vi "Periodic Tasks.vi"(0 "error in":errorcluster) -> ()   [LabVIEW 2020]
doc: "All TeleOperated, Autonomous, and Test controller logic are located here. Sensor reads and actuator commands are run inside of parallel loops. Most FRC 4265 code should be placed here."
uses:
  GlobalMiscellaneous.vi
  GlobalDriverStationData.vi
  GlobalAutonomous.vi
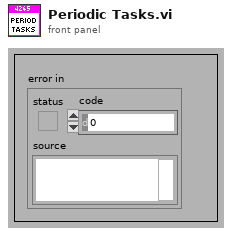
[diagram p1: front panel]
types:
  T1 = typedef "WPI_DriverStationRobotMode2.ctl" = enum16{"Autonomous Disabled", "Autonomous Enabled", "Teleop Disabled", "Teleop Enabled", "Disconnected", "Finish", "Test Disabled", "Test Enabled", "Emergency Stopped"}
  T2 = cluster{"Auto Error Out":errorcluster, "Drive Advance":bool, "Drive Step":i32, "Manipulator Step":i32, "Manipulator Advance":bool}
  T3 = cluster{"Auto Error":errorcluster, "Drive Advance":bool, "Drive Step":i32, "Manipulator Step":i32, "Manipulator Advance":bool}
  T4 = enum16{"Stowed", "Balancing", "Scoring", "Hoppering", "Ground", "Shelf"}
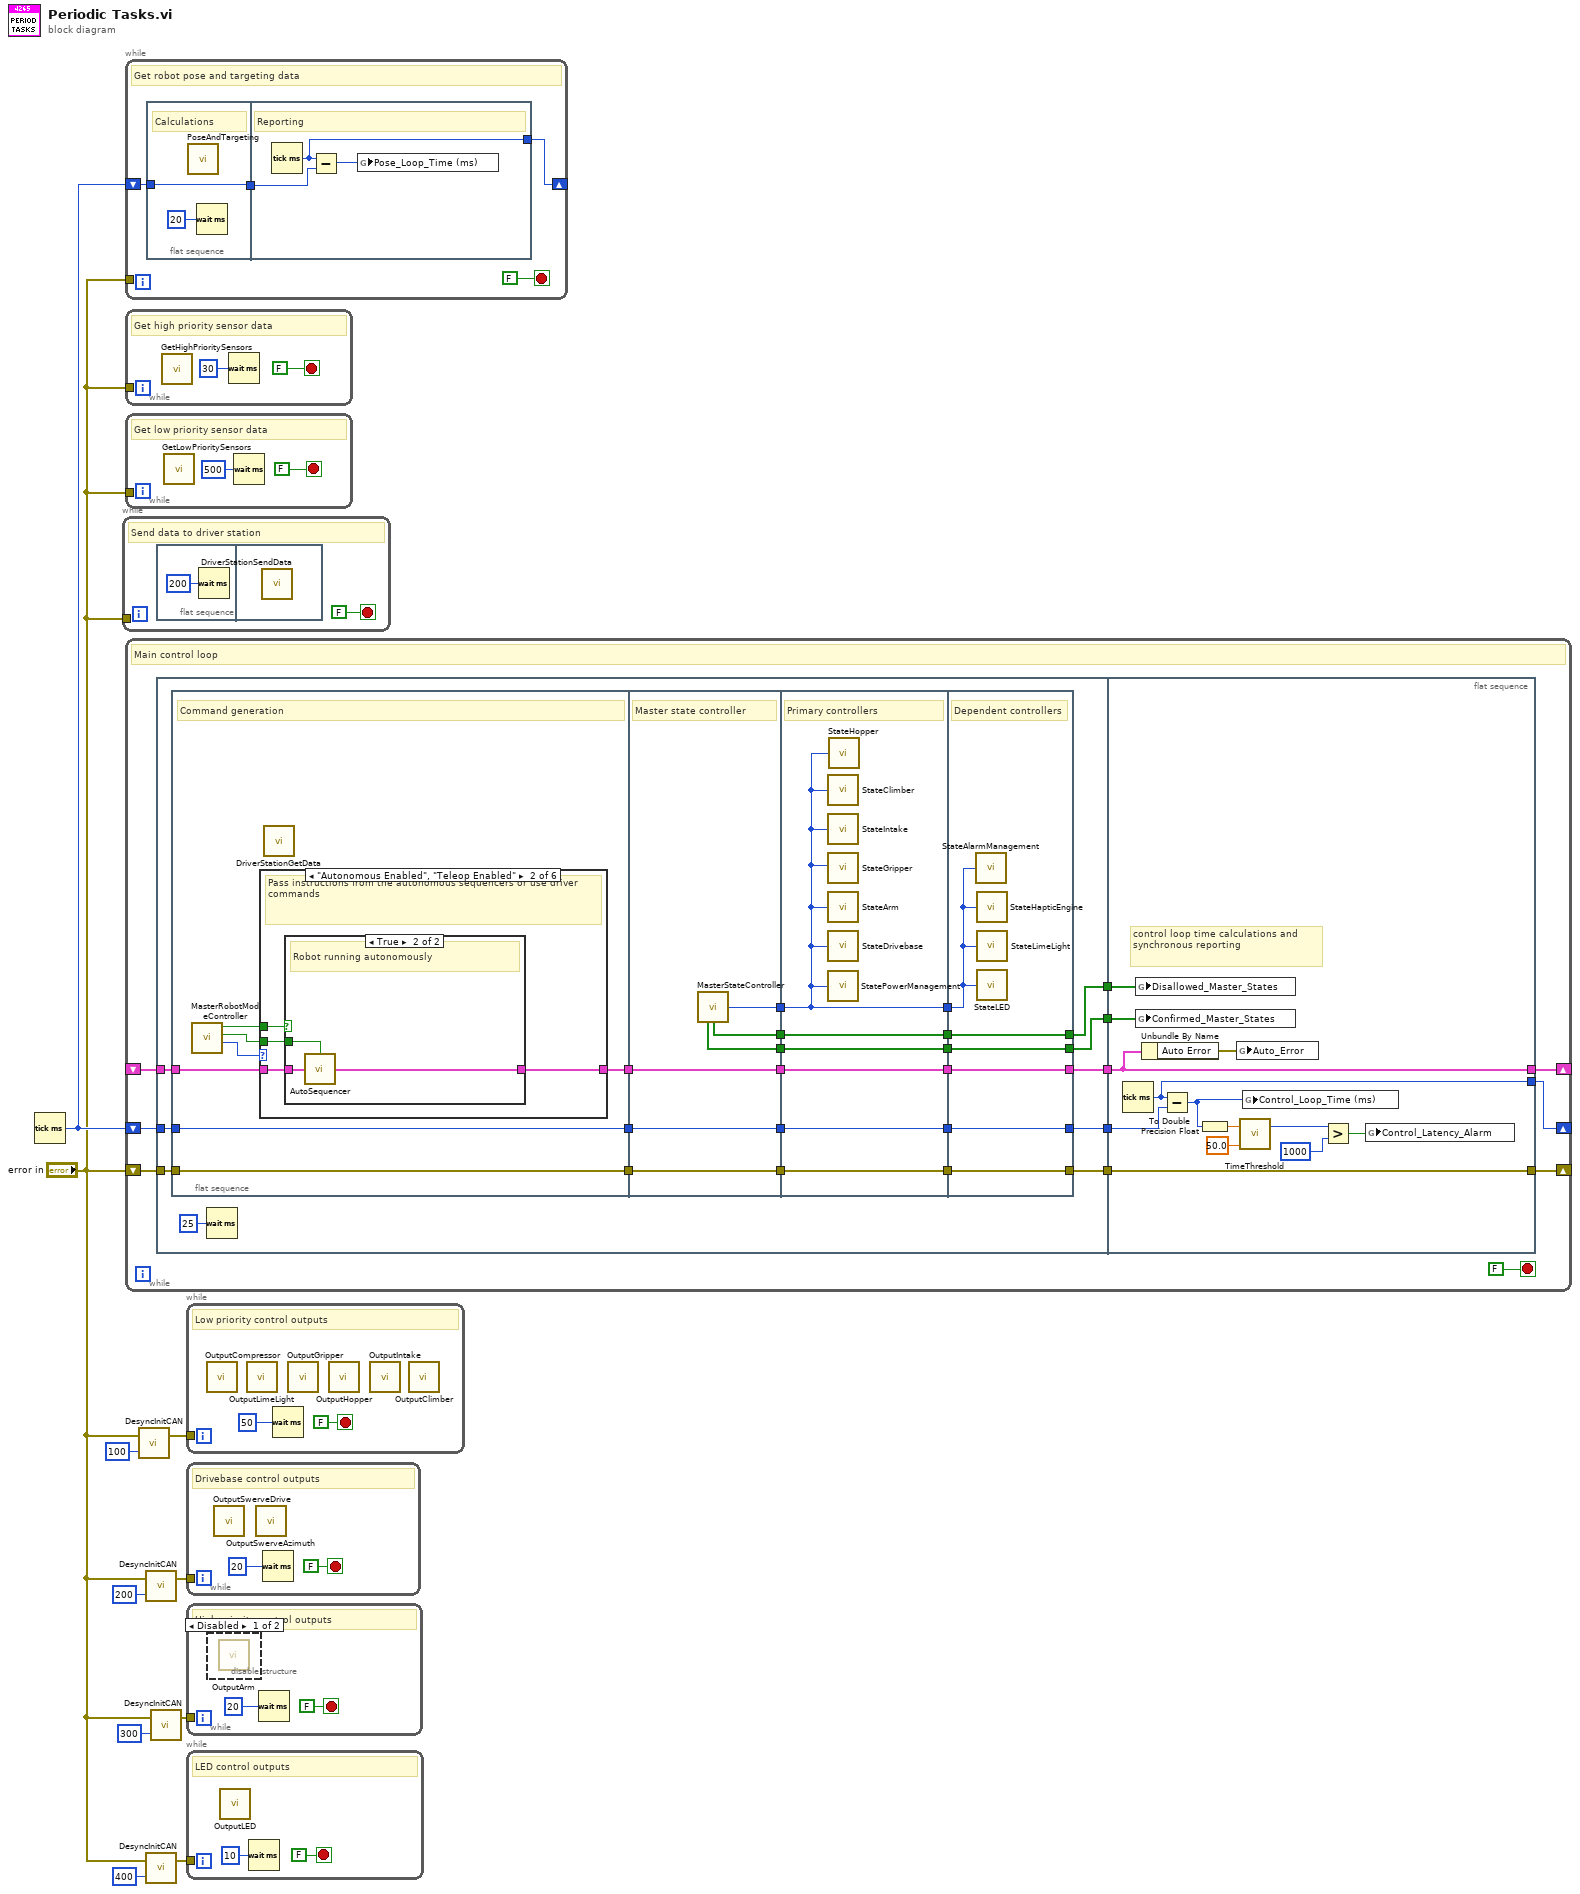
[diagram p0: block diagram]
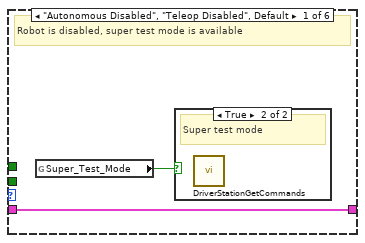
[diagram p3: hidden frame]
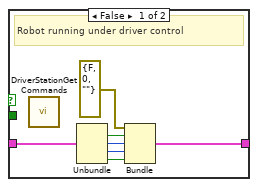
[diagram p5: hidden frame]
diagram:
  n1 = Tick Count (ms)() -> (millisecond timer value=w10:u32)
  n2 = while {
    tunnel: "error in" -> [_]
    stop <- FALSE stop-if-true
    # "Send data to driver station"
    n3 = flat-sequence {
      frame #0 {
        n4 = Wait (ms)(milliseconds to wait=u32 200) -> ()  [unwired: 1 out]
      }
      frame #1 {
        n5 = call "DriverStationSendData.vi"() -> ()  [unwired: 1 in]
      }
    }
  }
  n6 = while {
    tunnel: "error in" -> [_]
    shift-right: [w15] -> _
    shift-left: w10 -> [w14]
    stop <- FALSE stop-if-true
    # "Get robot pose and targeting data"
    n7 = flat-sequence {
      tunnel: w14 -> [w18]
      tunnel: [w18] -> w13
      tunnel: [w21] -> w15
      tunnel: w13 -> [w20]
      frame #0 {
        # "Calculations"
        n8 = call "PoseAndTargeting.vi"() -> ()  [unwired: 1 in]
        n9 = Wait (ms)(milliseconds to wait=u32 20) -> ()  [unwired: 1 out]
      }
      frame #1 {
        # "Reporting"
        n10 = Tick Count (ms)() -> (millisecond timer value=w21:u32)
        n11 = Subtract(x=w21, y=w20) -> (x-y=w19:u32)
        n12 = global write "GlobalMiscellaneous.vi" "Pose_Loop_Time (ms)"(w19) -> ()
      }
    }
  }
  n13 = while {
    tunnel: "error in" -> [_]
    stop <- FALSE stop-if-true
    # "Get high priority sensor data"
    n14 = call "GetHighPrioritySensors.vi"() -> ()  [unwired: 1 in]
    n15 = Wait (ms)(milliseconds to wait=u32 30) -> ()  [unwired: 1 out]
  }
  n16 = while {
    tunnel: "error in" -> [_]
    stop <- FALSE stop-if-true
    # "Get low priority sensor data"
    n17 = call "GetLowPrioritySensors.vi"() -> ()  [unwired: 1 in]
    n18 = Wait (ms)(milliseconds to wait=u32 500) -> ()  [unwired: 1 out]
  }
  n19 = while {
    shift-right: [w31] -> _
    shift-left: w10 -> [w32]
    shift-right: [w36] -> _
    shift-left: _ -> [w35]
    shift-right: [w33] -> _
    shift-left: "error in" -> [w34]
    stop <- FALSE stop-if-true
    # "Main control loop"
    n20 = flat-sequence {
      tunnel: w35 -> [w54]
      tunnel: w34 -> [w53]
      tunnel: w32 -> [w51]
      tunnel: [w55] -> w30
      tunnel: [w52] -> w29
      tunnel: [w49] -> w28
      tunnel: [w46] -> w27
      tunnel: [w44] -> w26
      tunnel: [w113] -> w31
      tunnel: [w119] -> w33
      tunnel: [w111] -> w36
      tunnel: w30 -> [w111]
      tunnel: w29 -> [w119]
      tunnel: w28 -> [w114]
      tunnel: w27 -> [w112]
      tunnel: w26 -> [w107]
      frame #0 {
        n21 = flat-sequence {
          tunnel: [w68] -> w61
          tunnel: w54 -> [w67]
          tunnel: [w63] -> w60
          tunnel: w53 -> [w63]
          tunnel: [w62] -> w59
          tunnel: w51 -> [w62]
          tunnel: [w94] -> w43
          tunnel: [w93] -> w42
          tunnel: w61 -> [w93]
          tunnel: w60 -> [w92]
          tunnel: [w92] -> w41
          tunnel: w59 -> [w91]
          tunnel: [w91] -> w40
          tunnel: [w90] -> w39
          tunnel: [w89] -> w38
          tunnel: w43 -> [w95]
          tunnel: [w100] -> w58
          tunnel: w42 -> [w100]
          tunnel: [w99] -> w57
          tunnel: w41 -> [w99]
          tunnel: [w98] -> w56
          tunnel: w40 -> [w98]
          tunnel: [w95] -> w48
          tunnel: [w97] -> w47
          tunnel: w39 -> [w97]
          tunnel: w38 -> [w96]
          tunnel: [w96] -> w45
          tunnel: [w106] -> w55
          tunnel: w58 -> [w106]
          tunnel: [w105] -> w52
          tunnel: w57 -> [w105]
          tunnel: w56 -> [w104]
          tunnel: [w104] -> w49
          tunnel: w48 -> [w102]
          tunnel: [w103] -> w46
          tunnel: w47 -> [w103]
          tunnel: w45 -> [w101]
          tunnel: [w101] -> w44
          frame #0 {
            # "Command generation"
            n22 = call "MasterRobotModeController.vi"() -> ("FMS Robot Mode"=w66:T1, "Auto Reset"=w65:bool, "Robot is Autonomous"=w64:bool)  [unwired: 5 in]
            n23 = case shown="\"Autonomous Enabled\", \"Teleop Enabled\"" w66 {
              tunnel: w65 -> [_ w72 _ _ _ _]
              tunnel: [w69 w74 w85 w86 w87 w88] -> w68
              tunnel: w67 -> [w69 w73 w85 w86 w87 w88]
              tunnel: w64 -> [_ w71 _ _ _ _]
              frame "Autonomous Disabled", "Teleop Disabled", Default {
                # "Robot is disabled, super test mode is available"
                n24 = global read "GlobalDriverStationData.vi" "Super_Test_Mode"() -> (w70:bool)
                n25 = case shown="True" w70 {
                  frame False {
                    # "Fully disabled"
                  }
                  frame True {
                    # "Super test mode"
                    n26 = call "DriverStationGetCommands.vi"() -> ()  [unwired: 12 in]
                  }
                }
              }
              frame "Autonomous Enabled", "Teleop Enabled" {
                # "Pass instructions from the autonomous sequencers or use driver commands"
                n27 = case shown="True" w71 {
                  tunnel: w72 -> [_ w84]
                  tunnel: [w80 w83] -> w74
                  tunnel: w73 -> [w81 w82]
                  frame False {
                    # "Robot running under driver control"
                    n28 = call "DriverStationGetCommands.vi"() -> ()  [unwired: 12 in]
                    n29 = Unbundle(w81) -> ("Drive Advance"=w76:bool, "Drive Step"=w77:i32, "Manipulator Step"=w78:i32, "Manipulator Advance"=w79:bool)  [unwired: 1 out]
                    n30 = Bundle("Auto Error Out"=errorcluster {"status"=FALSE, "code"=0, "source"=""}, "Drive Advance"=w76, "Drive Step"=w77, "Manipulator Step"=w78, "Manipulator Advance"=w79) -> (w80:T2)  [unwired: 1 in]
                  }
                  frame True {
                    # "Robot running autonomously"
                    n31 = call "AutoSequencer.vi"("Reinit Sequencer"=w84, "Auto Cluster In"=w82) -> ("Auto Cluster Out"=w83:T3)  [unwired: 13 in]
                  }
                }
              }
              frame "Finish" {
                # "Clean up operations are in the Finish.vi in RobotMain.vi"
              }
              frame "Test Disabled", "Test Enabled" {
                # "Use TestActuatorInterlock.vi for implimenting test code"
              }
              frame "Disconnected" {
                # "Communications have failed"
              }
              frame "Emergency Stopped" {
                # "Robot has been emergency stopped"
              }
            }
            n32 = call "DriverStationGetData.vi"() -> ()  [unwired: 1 in]
          }
          frame #1 {
            # "Master state controller"
            n33 = call "MasterStateController.vi"() -> ("Master State Out"=w94:T4, "Confirmed Master States"=w90:bool[], "Disallowed Master States"=w89:bool[])  [unwired: 13 in]
          }
          frame #2 {
            # "Primary controllers"
            n34 = call "StateClimber.vi"("Master State In"=w95) -> ()
            n35 = call "StateIntake.vi"("Master State In"=w95) -> ()
            n36 = call "StateGripper.vi"("Master State In"=w95) -> ()
            n37 = call "StateArm.vi"("Master State In"=w95) -> ()
            n38 = call "StateDrivebase.vi"("Master State In"=w95) -> ()
            n39 = call "StatePowerManagement.vi"("Master State In"=w95) -> ()
            n40 = call "StateHopper.vi"("Master State In"=w95) -> ()
          }
          frame #3 {
            # "Dependent controllers"
            n41 = call "StateAlarmManagement.vi"("Master State In"=w102) -> ()
            n42 = call "StateHapticEngine.vi"("Master State In"=w102) -> ()
            n43 = call "StateLimeLight.vi"("Master State In"=w102) -> ()
            n44 = call "StateLED.vi"("Master State In"=w102) -> ()
          }
        }
        n45 = Wait (ms)(milliseconds to wait=u32 25) -> ()  [unwired: 1 out]
      }
      frame #1 {
        # "control loop time calculations and synchronous reporting"
        n46 = Tick Count (ms)() -> (millisecond timer value=w113:u32)
        n47 = global write "GlobalMiscellaneous.vi" "Disallowed_Master_States"(w107) -> ()
        n48 = global write "GlobalMiscellaneous.vi" "Confirmed_Master_States"(w112) -> ()
        n49 = Unbundle By Name(w111) -> ("Auto Error"=w110:errorcluster)
        n50 = Subtract(x=w113, y=w114) -> (x-y=w109:u32)
        n51 = To Double Precision Float(number=w109) -> (double precision float=w118:dbl)
        n52 = global write "GlobalAutonomous.vi" "Auto_Error"(w110) -> ()
        n53 = call "TimeThreshold.vi"("Threshold"=50.0, "Current Value"=w118) -> ("Time Above Threshold (ms)"=w117:u32)  [unwired: 1 out]
        n54 = global write "GlobalMiscellaneous.vi" "Control_Loop_Time (ms)"(w109) -> ()
        n55 = Greater?(x=w117, y=u32 1000) -> (0:w108:bool)
        n56 = global write "GlobalMiscellaneous.vi" "Control_Latency_Alarm"(w108) -> ()
      }
    }
  }
  n57 = call "DesyncInitCAN.vi"("Desync Time (ms)"=u32 100, "error in"="error in") -> ("error out"=w9:errorcluster)  [unwired: 1 in]
  n58 = call "DesyncInitCAN.vi"("Desync Time (ms)"=u32 200, "error in"="error in") -> ("error out"=w6:errorcluster)  [unwired: 1 in]
  n59 = call "DesyncInitCAN.vi"("Desync Time (ms)"=u32 400, "error in"="error in") -> ("error out"=w2:errorcluster)  [unwired: 1 in]
  n60 = call "DesyncInitCAN.vi"("Desync Time (ms)"=u32 300, "error in"="error in") -> ("error out"=w4:errorcluster)  [unwired: 1 in]
  n61 = while {
    tunnel: w9 -> [_]
    stop <- FALSE stop-if-true
    # "Low priority control outputs"
    n62 = call "OutputCompressor.vi"() -> ()  [unwired: 1 in]
    n63 = call "OutputLimeLight.vi"() -> ()  [unwired: 1 in]
    n64 = Wait (ms)(milliseconds to wait=u32 50) -> ()  [unwired: 1 out]
    n65 = call "OutputGripper.vi"() -> ()  [unwired: 1 in]
    n66 = call "OutputHopper.vi"() -> ()  [unwired: 1 in]
    n67 = call "OutputIntake.vi"() -> ()  [unwired: 1 in]
    n68 = call "OutputClimber.vi"() -> ()  [unwired: 1 in]
  }
  n69 = while {
    tunnel: w6 -> [_]
    stop <- FALSE stop-if-true
    # "Drivebase control outputs"
    n70 = call "OutputSwerveDrive.vi"() -> ()  [unwired: 1 in]
    n71 = call "OutputSwerveAzimuth.vi"() -> ()  [unwired: 1 in]
    n72 = Wait (ms)(milliseconds to wait=u32 20) -> ()  [unwired: 1 out]
  }
  n73 = while {
    tunnel: w4 -> [_]
    stop <- FALSE stop-if-true
    # "High priority control outputs"
    n74 = disable-structure shown="Disabled" {
      frame Disabled {
        n75 = call "OutputArm.vi"() -> ()  [unwired: 1 in]
      }
      frame Enabled {
      }
    }
    n76 = Wait (ms)(milliseconds to wait=u32 20) -> ()  [unwired: 1 out]
  }
  n77 = while {
    tunnel: w2 -> [_]
    stop <- FALSE stop-if-true
    # "LED control outputs"
    n78 = call "OutputLED.vi"() -> ()  [unwired: 1 in]
    n79 = Wait (ms)(milliseconds to wait=u32 10) -> ()  [unwired: 1 out]
  }
